vi "Add Rx Frames.vi"(8 "error in (no error)":errorcluster, 10 "Frames":variant, 11 "CANBus_Load_Calculator in":refnum<class "CANBus_Load_Calculator.lvclass">) -> (0 "error out":errorcluster, 3 "CANBus_Load_Calculator out":refnum<class "CANBus_Load_Calculator.lvclass">)   [LabVIEW 2019, in "XNET-Bus-Load-Calculator.lvlib" / "CANBus_Load_Calculator.lvclass"]
uses:
  CANBus_Load_Calculator.lvclass
  C:/Users/angomez/Documents/GitHub/XNET-Bus-Load-Calculator/GenBus/GenBus_Load_Calculator.lvclass
  GenBus/GenBus_Load_Calculator.lvclass/GenBus_Load_Calculator.ctl
  <vilib>/xnet/xnet.llb/XNET Frame CAN.ctl
  <vilib>/xnet/xnet.llb/XNET Frame Type CAN.ctl
  GenBus/GenBus_Load_Calculator.lvclass
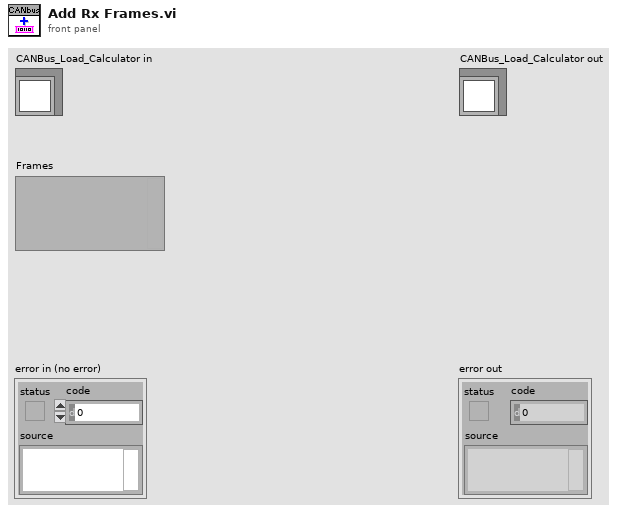
[diagram p1: front panel]
types:
  T1 = typedef "XNET Frame CAN.ctl" = cluster{"timestamp":timestamp, "payload":u8[], "identifier":u32, "type":T2, "extended?":bool, "echo?":bool}
  T2 = typedef "XNET Frame Type CAN.ctl" = u8
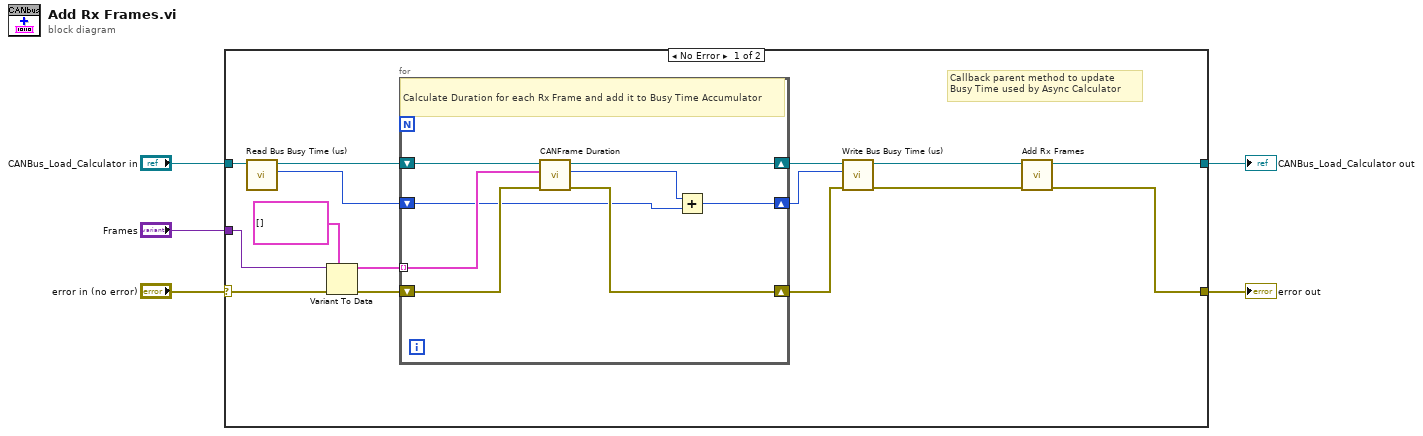
[diagram p0: block diagram]
diagram:
  n1 = case shown="No Error" "error in (no error)" {
    selector: "error in (no error)" -> [w20 w30]
    tunnel: [w6 w30] -> w4
    tunnel: [w8 w29] -> w1
    tunnel: "CANBus_Load_Calculator in" -> [w15 w29]
    tunnel: "Frames" -> [w18 _]
    frame No Error {
      # "Callback parent method to update\nBusy Time used by Async Calculator"
      n2 = call "Read Bus Busy Time (us).vi"("GenBus_Load_Calculator in"=w15) -> ("Bus Busy Time (us)"=w12:u64, "GenBus_Load_Calculator out"=w10:refnum<class "CANBus_Load_Calculator.lvclass">)  [unwired: 8 in, 1 out]
      n3 = Variant To Data(error in=w20, type=T1[] [] ("CAN Frames"), Variant=w18) -> (data=w16:T1[], error out=w17:errorcluster)
      n4 = for {
        tunnel: w16 -> [w28] mode=indexing
        shift-right: [w27] -> w13
        shift-left: w17 -> [w26]
        shift-right: [w21] -> w11
        shift-left: w12 -> [w22]
        shift-right: [w25] -> w9
        shift-left: w10 -> [w24]
        # "Calculate Duration for each Rx Frame and add it to Busy Time Accumulator"
        n5 = call "CANFrame Duration.vi"("error in (no error)"=w26, "CAN frame"=w28, "CANBus_Load_Calculator in"=w24) -> ("error out"=w27:errorcluster, "Frame Duration (us)"=w23:u64, "CANBus_Load_Calculator out"=w25:refnum<class "CANBus_Load_Calculator.lvclass">)  [unwired: 6 in]
        n6 = Add(x=w23, y=w22) -> (x+y=w21:u64)
      }
      n7 = call "Write Bus Busy Time (us).vi"("error in (no error)"=w13, "Bus Busy Time (us)"=w11, "GenBus_Load_Calculator in"=w9) -> ("error out"=w7:errorcluster, "GenBus_Load_Calculator out"=w14:refnum<class "CANBus_Load_Calculator.lvclass">)  [unwired: 7 in]
      n8 = call-parent "Add Rx Frames.vi"("error in (no error)"=w7, "GenBus_Load_Calculator in"=w14) -> ("error out"=w6:errorcluster, "GenBus_Load_Calculator out"=w8:refnum<class "CANBus_Load_Calculator.lvclass">)  [unwired: 8 in]
    }
    frame Error {
    }
  }
  "error out" <- w4
  "CANBus_Load_Calculator out" <- w1
